vi "CSM - Filter Sync Messages.vi"(5 "State(s) in (\"\")":string) -> (6 "States Out":string)   [LabVIEW 2017, in "Communicable State Machine.lvlib"]
doc: "Filter messages sent to non-existing modules.\nThis VI uses CSM - List Modules.vi to get all active CSM modules and then filters out messages sent to non-existing modules.\n\n-- <b>Controls</b> --\n- <b>States</b>: Input message string\n\n-- <b>Indicators</b> --\n- <b>Filtered States</b>: Filtered message string"
uses:
  _Support/Common/Trim Single line Text.vi
  Communicable State Machine.lvlib
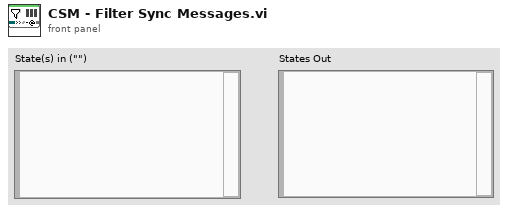
[diagram p1: front panel]
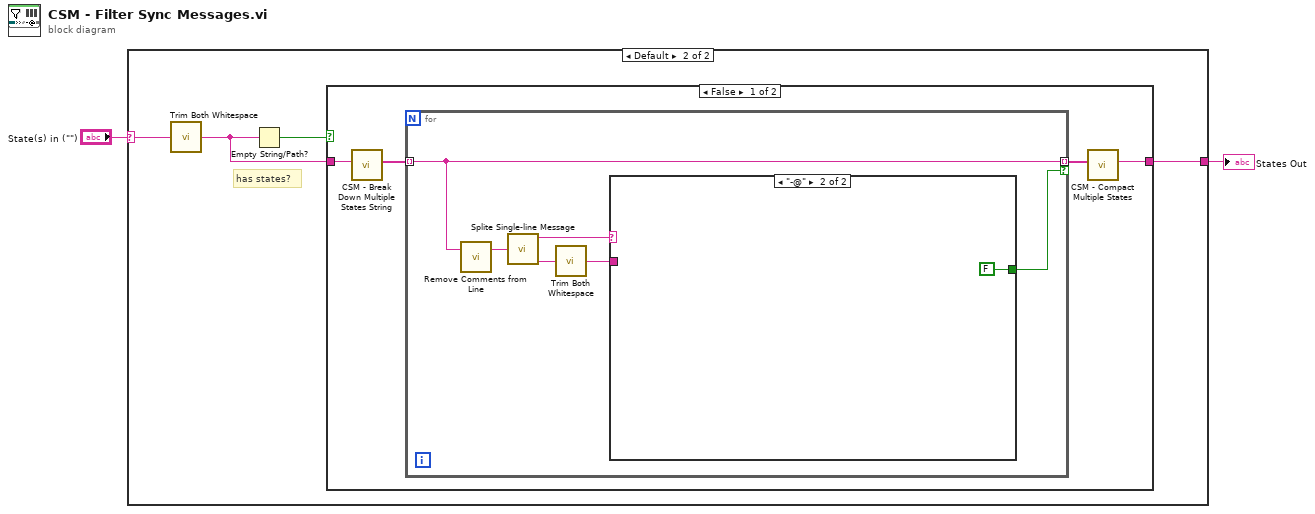
[diagram p0: block diagram]
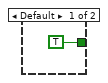
[diagram p3: hidden frame]
diagram:
  n1 = case shown="Default" "State(s) in (\"\")" {
    selector: "State(s) in (\"\")" -> [_ w3]
    tunnel: [_ w6] -> w1
    frame "" {
    }
    frame Default {
      # "has states?"
      n2 = call "Trim Both Whitespace.vi"("string"=w3) -> ("trimmed string"=w4:string)  [unwired: 1 in]
      n3 = Empty String/Path?(string/path=w4) -> (empty?=w5:bool)
      n4 = case shown="False" w5 {
        tunnel: w4 -> [w10 w19]
        tunnel: [w9 w19] -> w6
        frame False {
          n5 = call "CSM - Break Down Multiple States String.vi"("States"=w10) -> ("Multiple States"=w8:string[])  [unwired: 10 in]
          n6 = for {
            tunnel: w8 -> [w15] mode=indexing
            tunnel: [w15] -> w7 mode=indexing if=w13
            n7 = call "Remove Comments from Line.vi"("single-line text"=w15) -> ("single-line text without comments"=w16:string)  [unwired: 2 in]
            n8 = call "Splite Single-line Message.vi"("single-line text"=w16) -> ("operator"=w14:string, "source/target"=w12:string)  [unwired: 6 in, 2 out]
            n9 = call "Trim Both Whitespace.vi"("string"=w12) -> ("trimmed string"=w11:string)  [unwired: 1 in]
            n10 = case shown="\"-@\"" w14 {
              tunnel: [TRUE FALSE] -> w13
              tunnel: w11 -> [_ _]
              frame Default {
              }
              frame "-@" {
              }
            }
          }
          n11 = call "CSM - Compact Multiple States.vi"("Multiple States"=w7) -> ("States"=w9:string)  [unwired: 9 in]
        }
        frame True {
        }
      }
    }
  }
  "States Out" <- w1
